vi "TCP Client.vi"() -> ()   [LabVIEW 2021]
doc: "The myRIO Project template acquires acceleration data from the onboard accelerometer and displays the changes of acceleration values in a waveform chart."
panel:
  out "error out":errorcluster
  in  "Port":u16
  in  "Address":string
  out "Received":string
  in  "Payload":string
  in  "Connect":bool
  in  "Send":bool
  out "Connected":bool
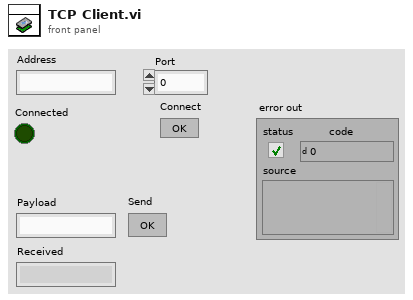
[diagram p1: front panel]
types:
  T1 = enum16{"Start Opening", "Opening", "Start Connecting", "Connected", "Disconnected"}
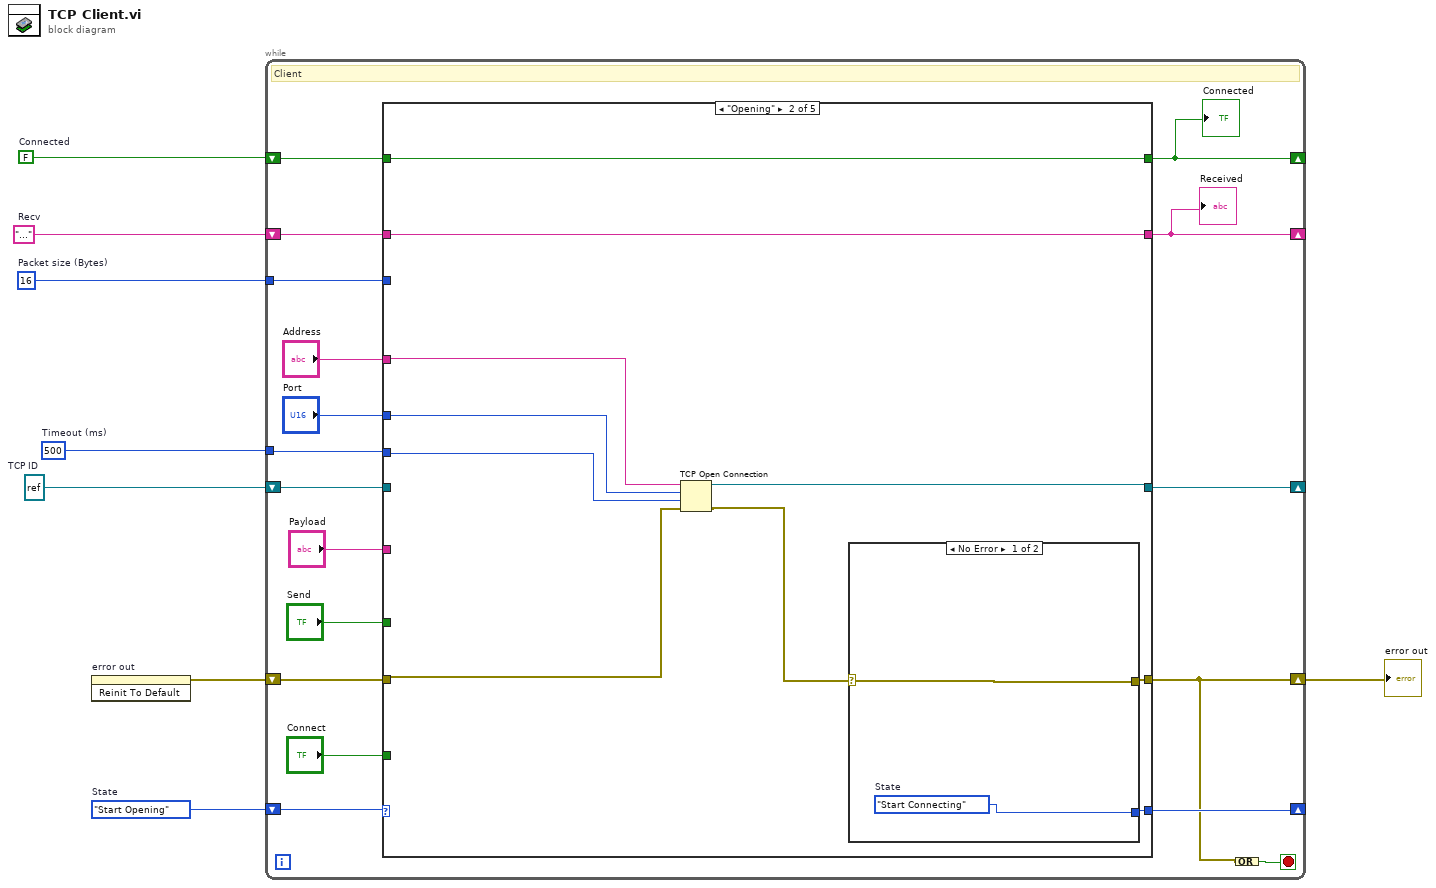
[diagram p0: block diagram]
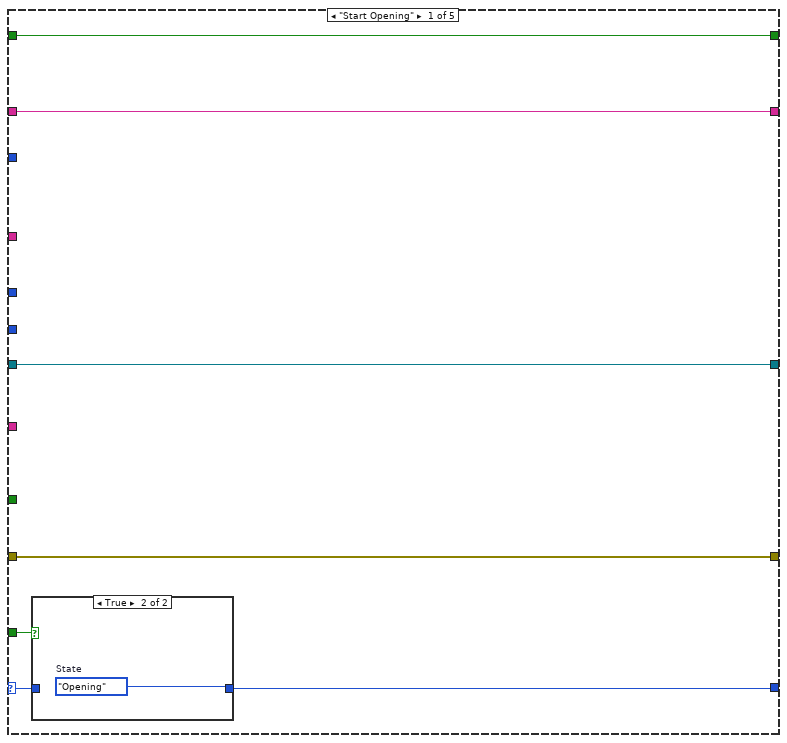
[diagram p2: hidden frame]
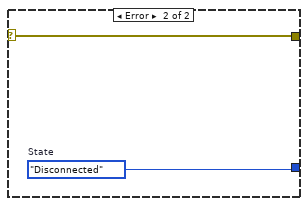
[diagram p4: hidden frame]
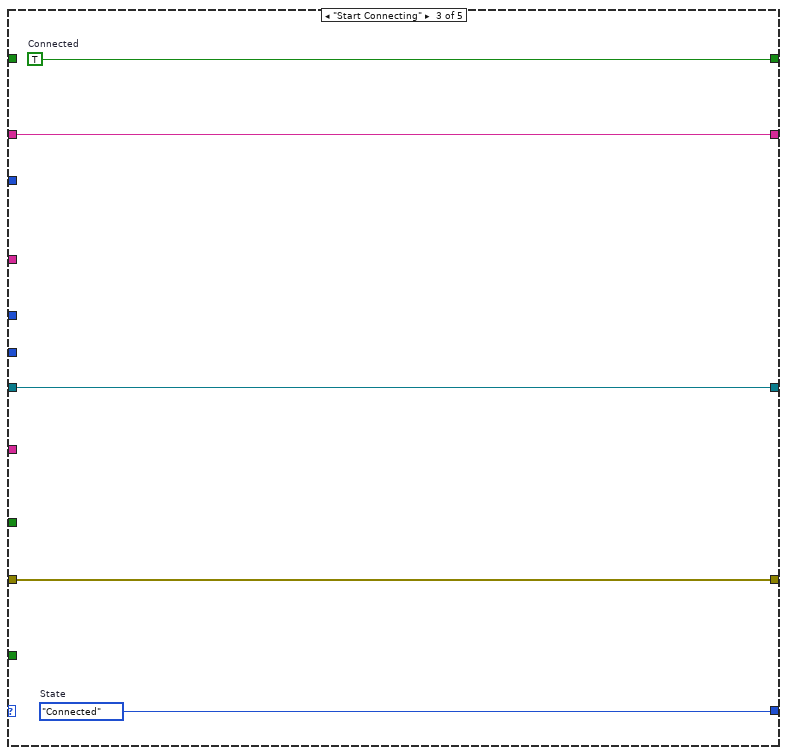
[diagram p5: hidden frame]
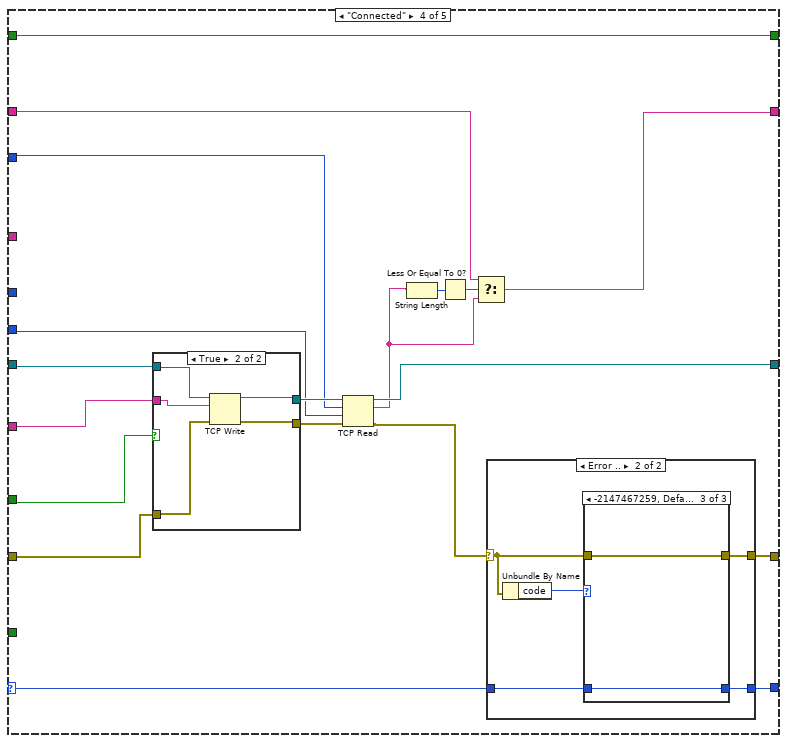
[diagram p6: hidden frame]
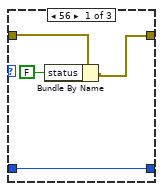
[diagram p8: hidden frame]
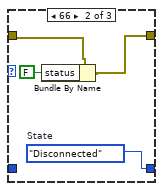
[diagram p9: hidden frame]
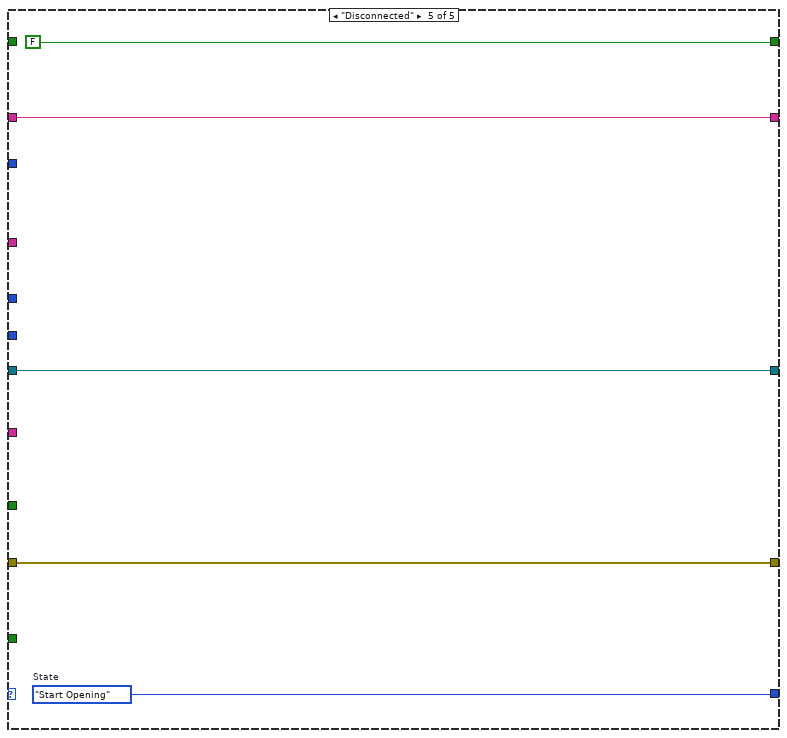
[diagram p11: hidden frame]
diagram:
  w6 = refnum<k5> refnum  # TCP ID
  w5 = 500  # Timeout (ms)
  w4 = 16  # Packet size (Bytes)
  w3 = "..."  # Recv
  w2 = FALSE  # Connected
  w8 = T1."Start Opening"  # State
  n1 = invoke on="error out" class="Clust (strict)" method="Reinit To Default"() -> (error out=w7:errorcluster)  [unwired: 3 in, 2 out]
  n2 = while {
    tunnel: w5 -> [w19]
    tunnel: w4 -> [w17]
    shift-right: [w11] -> _
    shift-left: w8 -> [w26]
    shift-right: [w10] -> w1
    shift-left: w7 -> [w24]
    shift-right: [w12] -> _
    shift-left: w6 -> [w18]
    shift-right: [w13] -> _
    shift-left: w2 -> [w15]
    shift-right: [w14] -> _
    shift-left: w3 -> [w16]
    stop <- w9 stop-if-true
    # "Client"
    n3 = case shown="\"Opening\"" w26 {
      selector: w26 -> [w32 _ _ w57 _]
      tunnel: "Connect" -> [w33 _ _ _ _]
      tunnel: w24 -> [w27 w40 w51 w68 w99]
      tunnel: "Send" -> [_ _ _ w71 _]
      tunnel: "Payload" -> [_ _ _ w69 _]
      tunnel: "Port" -> [_ w42 _ _ _]
      tunnel: "Address" -> [_ w43 _ _ _]
      tunnel: w19 -> [_ w41 _ w65 _]
      tunnel: w18 -> [w29 _ w52 w70 w100]
      tunnel: w17 -> [_ _ _ w64 _]
      tunnel: w16 -> [w30 w44 w53 w61 w101]
      tunnel: w15 -> [w31 w45 _ w59 _]
      tunnel: [w31 w45 w54 w59 FALSE] -> w13
      tunnel: [w30 w44 w53 w60 w101] -> w14
      tunnel: [w29 w39 w52 w63 w100] -> w12
      tunnel: [w28 w36 w50 w56 w98] -> w11
      tunnel: [w27 w37 w51 w55 w99] -> w10
      frame "Start Opening" {
        n4 = case shown="True" w33 {
          tunnel: w32 -> [w34 _]
          tunnel: [w34 w35] -> w28
          frame False {
          }
          frame True {
            w35 = T1."Opening"  # State
          }
        }
      }
      frame "Opening" {
        n5 = TCP Open Connection(address=w43, remote port or service name=w42, timeout ms (60000)=w41, error in (no error)=w40) -> (connection ID=w39:refnum<k5>, error out=w38:errorcluster)  [unwired: 1 in]
        n6 = case shown="No Error" w38 {
          selector: w38 -> [w47 w49]
          tunnel: [w47 w49] -> w37
          tunnel: [w46 w48] -> w36
          frame No Error {
            w46 = T1."Start Connecting"  # State
          }
          frame Error {
            w48 = T1."Disconnected"  # State
          }
        }
      }
      frame "Start Connecting" {
        w50 = T1."Connected"  # State
        w54 = TRUE  # Connected
      }
      frame "Connected" {
        n7 = case shown="True" w71 {
          tunnel: w70 -> [w92 w97]
          tunnel: w69 -> [_ w95]
          tunnel: w68 -> [w91 w94]
          tunnel: [w92 w96] -> w67
          tunnel: [w91 w93] -> w66
          frame False {
          }
          frame True {
            n8 = TCP Write(connection ID=w97, data in=w95, error in (no error)=w94) -> (connection ID out=w96:refnum<k5>, error out=w93:errorcluster)  [unwired: 1 in, 1 out]
          }
        }
        n9 = TCP Read(connection ID=w67, bytes to read=w64, error in (no error)=w66, 9:w65) -> (connection ID out=w63:refnum<k5>, data out=w62:string, error out=w58:errorcluster)  [unwired: 1 in]
        n10 = String Length(string=w62) -> (length=w72:i32)
        n11 = Less Or Equal To 0?(x=w72) -> (x <= 0?=w73:bool)
        n12 = Select(t=w61, s=w73, f=w62) -> (s? t:f=w60:string)
        n13 = case shown="Error .." w58 {
          selector: w58 -> [w74 w80]
          tunnel: w57 -> [w75 w77]
          tunnel: [w75 w76] -> w56
          tunnel: [w74 w78] -> w55
          frame No Error {
          }
          frame Error {
            n14 = Unbundle By Name(w80) -> ("code"=w79:i32)
            n15 = case shown="-2147467259, Default" w79 {
              tunnel: w80 -> [w83 w87 w90]
              tunnel: [w82 w86 w90] -> w78
              tunnel: w77 -> [w81 _ w89]
              tunnel: [w81 w85 w89] -> w76
              frame 56 {
                n16 = Bundle By Name(cluster=w83, "status"=FALSE) -> (w82:errorcluster)
              }
              frame 66 {
                w85 = T1."Disconnected"  # State
                n17 = Bundle By Name(cluster=w87, "status"=FALSE) -> (w86:errorcluster)
              }
              frame -2147467259, Default {
              }
            }
          }
        }
      }
      frame "Disconnected" {
        w98 = T1."Start Opening"  # State
      }
    }
    "Connected" <- w13
    "Received" <- w14
    n18 = Compound Arithmetic op=OR(w10) -> (w9:bool)
  }
  "error out" <- w1
